vi "Force mapping VI.vi"() -> ()   [LabVIEW 2017]
uses:
  <vilib>/Analysis/baseanly.llb/A x Vector.vi
  <vilib>/Analysis/NI_AALBase.lvlib
panel:
  in  "file path (dialog if empty)":path=path "C:/Users/FEEStaff/Documents/Wind Tunnel Results/RawData/Liebeck L1003 Dry Test 1_1"
  out "Lift":cluster{i32[], dbl[]}(graph)
  out "Drag":cluster{i32[], dbl[]}(graph)
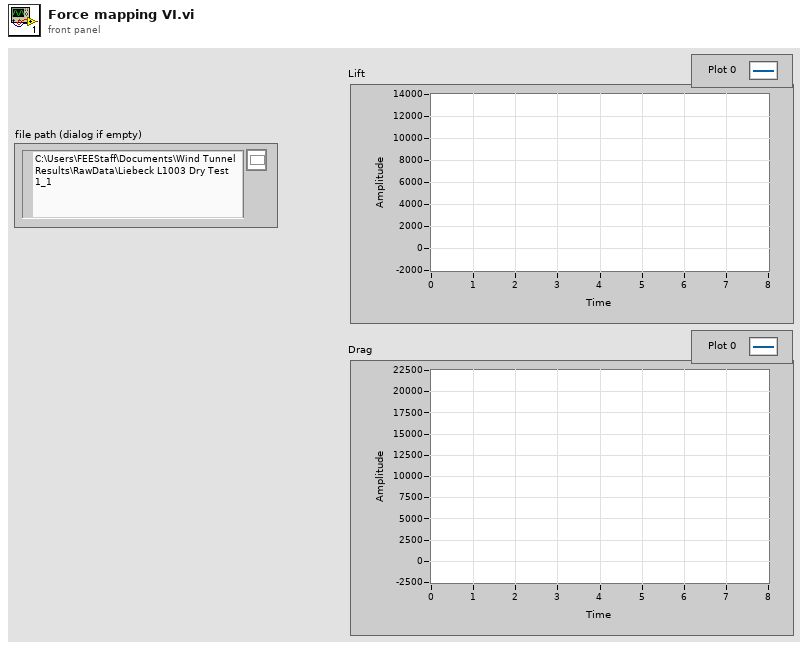
[diagram p1: front panel]
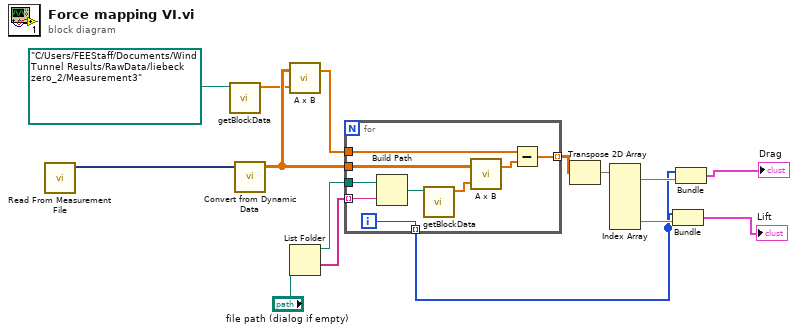
[diagram p0: block diagram]
diagram:
  n1 = call "Read From Measurement File"() -> ("Signals"=w12:dynamicdata)  [unwired: 6 in, 5 out]
  n2 = call "getBlockData.vi"("path in"=path "C:/Users/FEEStaff/Documents/Wind Tunnel Results/RawData/liebeck zero_2/Measurement3" ("file path (dialog if empty)")) -> ("Array"=w10:dbl[])  [unwired: 9 in, 1 out]
  n3 = call "Convert from Dynamic Data"("Dynamic Data Type"=w12) -> ("Array"=w11:dbl[][])  [unwired: 3 in]
  n4 = call-poly <vilib>:"A x B.vi"("Vector"=w10, "A"=w11) -> ("A x Vector"=w8:dbl[])  [unwired: 1 out]
  n5 = List Folder(path="file path (dialog if empty)") -> (path out=w14:path, folder names=w13:string[])  [unwired: 3 in, 2 out]
  n6 = for {
    tunnel: w14 -> [w24]
    tunnel: w13 -> [w23] mode=indexing
    tunnel: w11 -> [w22]
    tunnel: w8 -> [w19]
    tunnel: [w17] -> w7 mode=indexing
    tunnel: [w16] -> w2 mode=indexing
    i -> [w16]
    n7 = Build Path(base path=w24, name or relative path=w23) -> (appended path=w20:path)
    n8 = call "getBlockData.vi"("path in"=w20) -> ("Array"=w21:dbl[])  [unwired: 9 in, 1 out]
    n9 = call-poly <vilib>:"A x B.vi"("Vector"=w21, "A"=w22) -> ("A x Vector"=w18:dbl[])  [unwired: 1 out]
    n10 = Subtract(x=w19, y=w18) -> (x-y=w17:dbl[])
  }
  n11 = Transpose 2D Array(2D array=w7) -> (transposed array=w1:dbl[][])
  n12 = Index Array(array=w1) -> (element #1=w4:dbl[], element #3=w3:dbl[])  [unwired: 6 in, 1 out]
  n13 = Bundle(w2, w3) -> (→"Lift":cluster{i32[], dbl[]})  [unwired: 1 in]
  n14 = Bundle(w2, w4) -> (→"Drag":cluster{i32[], dbl[]})  [unwired: 1 in]
